vi "main.vi"   [LabVIEW 2023]
types:
  T1 = enum16{"Left Button", "Center Button", "Right Button", "Window Close"}
  T2 = enum32{"Invalid", "Standard", "Closed", "Hidden", "Minimized", "Maximized"}
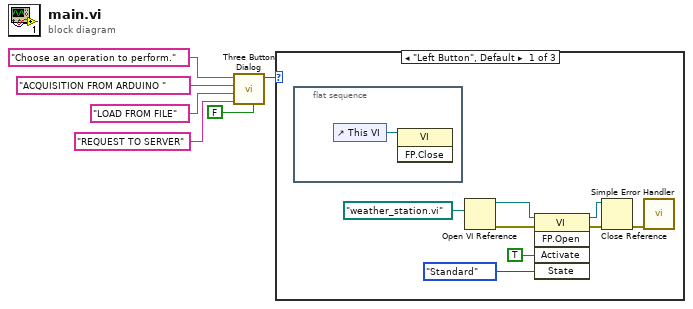
[diagram p0: block diagram]
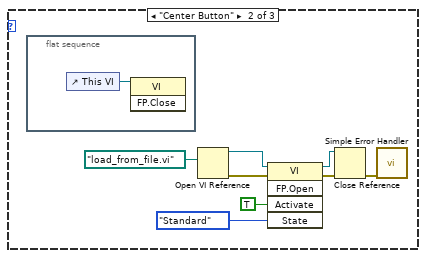
[diagram p2: hidden frame]
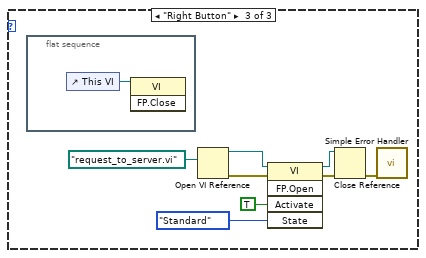
[diagram p3: hidden frame]
diagram:
  n1 = call <vilib>:"Three Button Dialog.vi"("Allow user to close window? (TRUE)"=FALSE, "Right Button Text (\"Cancel\")"="REQUEST TO SERVER" ("Right Button Text (\"Cancel\")"), "Center Button Text (\"No\")"="LOAD FROM FILE" ("Center Button Text (\"No\")"), "Left Button Text (\"Yes\")"="ACQUISITION FROM ARDUINO " ("Left Button Text (\"Yes\")"), "message"="Choose an operation to perform.") -> ("Which Button?"=w2:T1)  [unwired: 6 in]
  n2 = case shown="\"Left Button\", Default" w2 {
    frame "Left Button", Default {
      n3 = flat-sequence {
        frame #0 {
          n4 = control-ref of="This VI"() -> (w15:refnum<vi>)
          n5 = invoke class="VI" method="FP.Close"(reference=w15) -> ()  [unwired: 2 in, 3 out]
        }
      }
      n6 = Open VI Reference(vi path=path "weather_station.vi") -> (vi reference=w12:refnum<vi>, error out=w11:errorcluster)  [unwired: 5 in]
      n7 = invoke class="VI" method="FP.Open"(reference=w12, error in=w11, "Activate"=TRUE ("Activate?"), "State"=T2."Standard") -> (reference out=w8:refnum<vi>, error out=w7:errorcluster)  [unwired: 1 in, 3 out]
      n8 = Close Reference(reference=w8, error in (no error)=w7) -> (error out=w14:errorcluster)
      n9 = call <vilib>:"Simple Error Handler.vi"("error in (no error)"=w14) -> ()  [unwired: 4 in, 5 out]
    }
    frame "Center Button" {
      n10 = flat-sequence {
        frame #0 {
          n11 = control-ref of="This VI"() -> (w24:refnum<vi>)
          n12 = invoke class="VI" method="FP.Close"(reference=w24) -> ()  [unwired: 2 in, 3 out]
        }
      }
      n13 = Open VI Reference(vi path=path "load_from_file.vi") -> (vi reference=w21:refnum<vi>, error out=w22:errorcluster)  [unwired: 5 in]
      n14 = invoke class="VI" method="FP.Open"(reference=w21, error in=w22, "Activate"=TRUE ("Activate?"), "State"=T2."Standard") -> (reference out=w17:refnum<vi>, error out=w16:errorcluster)  [unwired: 1 in, 3 out]
      n15 = Close Reference(reference=w17, error in (no error)=w16) -> (error out=w23:errorcluster)
      n16 = call <vilib>:"Simple Error Handler.vi"("error in (no error)"=w23) -> ()  [unwired: 4 in, 5 out]
    }
    frame "Right Button" {
      n17 = flat-sequence {
        frame #0 {
          n18 = control-ref of="This VI"() -> (w33:refnum<vi>)
          n19 = invoke class="VI" method="FP.Close"(reference=w33) -> ()  [unwired: 2 in, 3 out]
        }
      }
      n20 = Open VI Reference(vi path=path "request_to_server.vi") -> (vi reference=w30:refnum<vi>, error out=w31:errorcluster)  [unwired: 5 in]
      n21 = invoke class="VI" method="FP.Open"(reference=w30, error in=w31, "Activate"=TRUE ("Activate?"), "State"=T2."Standard") -> (reference out=w26:refnum<vi>, error out=w25:errorcluster)  [unwired: 1 in, 3 out]
      n22 = Close Reference(reference=w26, error in (no error)=w25) -> (error out=w32:errorcluster)
      n23 = call <vilib>:"Simple Error Handler.vi"("error in (no error)"=w32) -> ()  [unwired: 4 in, 5 out]
    }
  }
